vi "Raport USB.vi"(11 "error in (no error)":errorcluster) -> (4 "Komunikat":string="Brak połaczenia z urządzeniem,\nProblem komunikacyjny z USB\nSprawdź kabel lub gniazdo", 6 "USB?":bool)   [LabVIEW 2014]
doc: "Sprawdza czy błąd w klastrze \nma numes związany z obsługą USB\njesli tak to zgłasza komunikat"
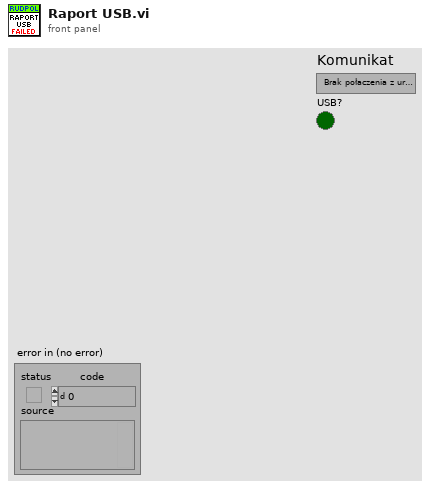
[diagram p1: front panel]
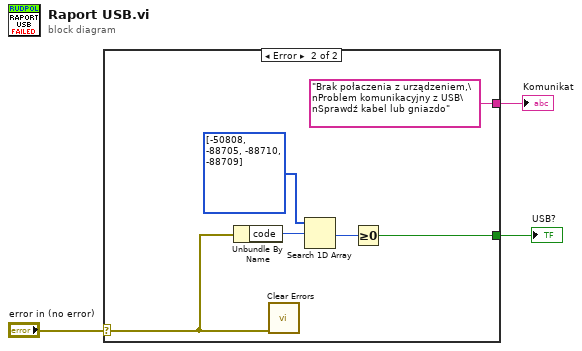
[diagram p0: block diagram]
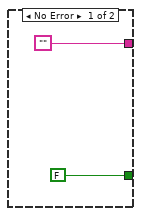
[diagram p2: hidden frame]
diagram:
  n1 = case shown="Error" "error in (no error)" {
    selector: "error in (no error)" -> [_ w6]
    tunnel: [FALSE w8] -> w2
    tunnel: ["" "Brak połaczenia z urządzeniem,\nProblem komunikacyjny z USB\nSprawdź kabel lub gniazdo"] -> w1
    frame No Error {
    }
    frame Error {
      n2 = Unbundle By Name(w6) -> ("code"=w10:i32)
      n3 = call <vilib>:"Clear Errors.vi"("error in (no error)"=w6) -> ()  [unwired: 5 in, 2 out]
      n4 = Search 1D Array(1D array=i32[] [-50808, -88705, -88710, -88709], element=w10) -> (index of element=w9:i32)  [unwired: 1 in]
      n5 = Greater Or Equal To 0?(x=w9) -> (x >= 0?=w8:bool)
    }
  }
  "USB?" <- w2
  "Komunikat" <- w1
